vi "Main - Fan Characterisation - Dynamic - [Student].vi"() -> ()   [LabVIEW 2017]
uses:
  <vilib>/Utility/file.llb/Read Delimited Spreadsheet (DBL).vi
  <vilib>/Analysis/baseanly.llb/Mean (DBL).vi
  <vilib>/Utility/file.llb/Write To Spreadsheet File (DBL).vi
  <vilib>/Analysis/NI_AALPro.lvlib
  <vilib>/Analysis/NI_AALBase.lvlib
panel:
  out "Post Processed Output":dbl[][](graph)
  out "Run-Time Data":cluster{"f":dbl, dbl}(graph)
  out "Time (s)":dbl(slide) scale=0.0..10.0
  out "Load Cell Calibration Data":cluster{"Y":dbl[], "Y":dbl[]}[](graph)
  in  "stop":bool
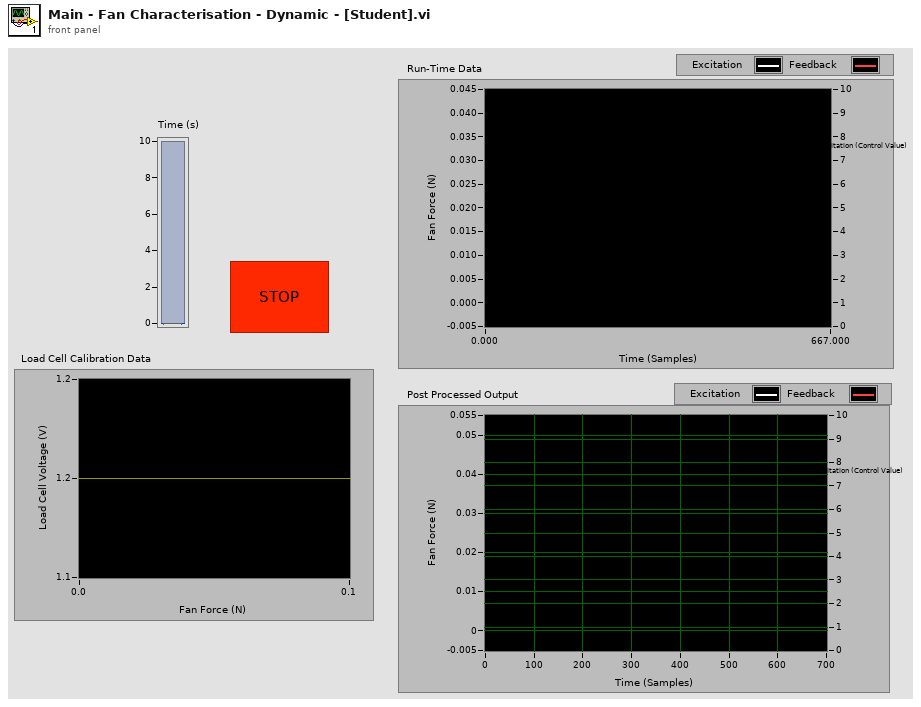
[diagram p1: front panel]
types:
  T1 = cluster{"AI Task":refnum<k21>, "Ctr0 Task":refnum<k21>, "Ao Task":refnum<k21>, "DO Task":refnum<k21>}
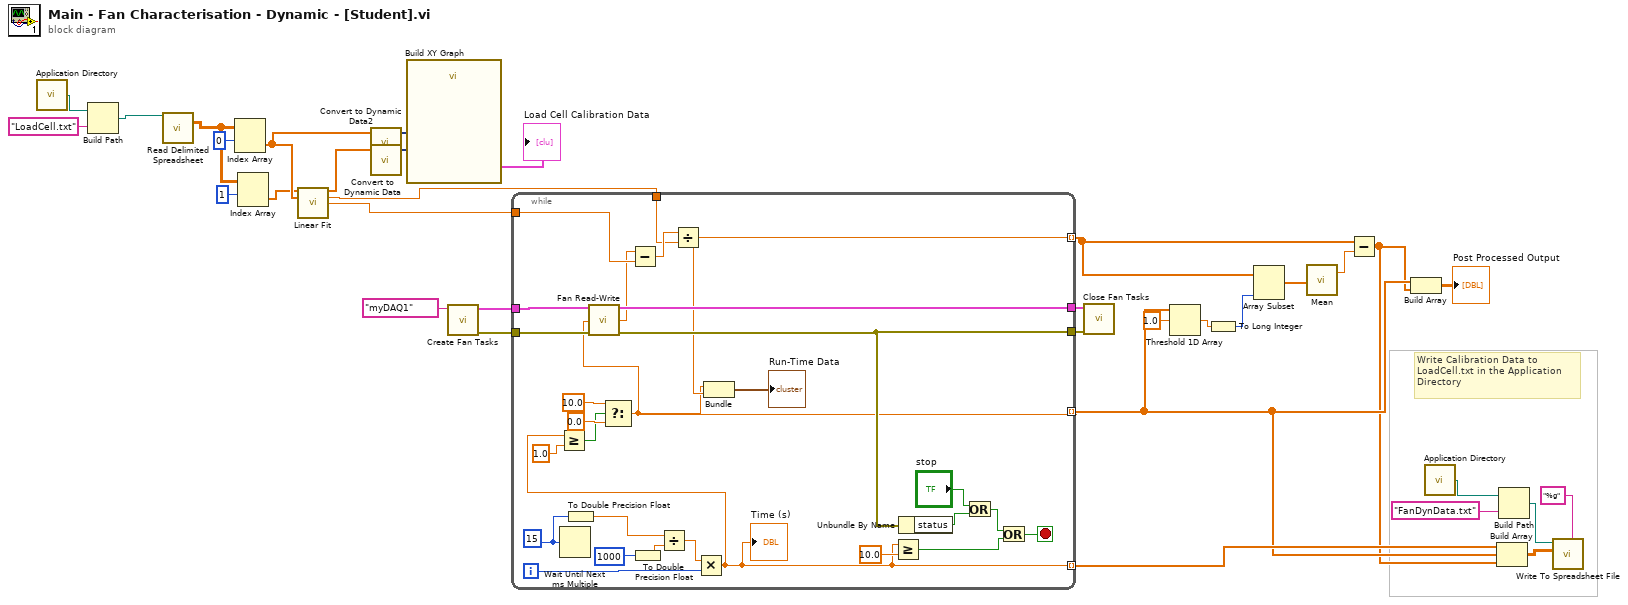
[diagram p0: block diagram]
diagram:
  # "Write Calibration Data to \nLoadCell.txt in the Application \nDirectory"
  n1 = call <vilib>:"Application Directory.vi"() -> ("Application Directory"=w23:path)
  n2 = Build Path(base path=w23, name or relative path="LoadCell.txt") -> (appended path=w22:path)
  n3 = call-poly <vilib>:"Read Delimited Spreadsheet.vi"("file path (dialog if empty)"=w22) -> ("all rows"=w25:dbl[][])  [unwired: 9 in, 5 out]
  n4 = Index Array(array=w25, index (row)=0) -> (element=w28:dbl[])  [unwired: 1 in]
  n5 = Index Array(array=w25, index (row)=1) -> (element=w26:dbl[])  [unwired: 1 in]
  n6 = call <vilib>:"Linear Fit.vi"("Y"=w26, "X"=w28) -> ("Best Linear Fit"=w16:dbl[], "slope"=w17:dbl, "intercept"=w18:dbl)  [unwired: 9 in, 2 out]
  n7 = call "Convert to Dynamic Data2"("Array"=w28) -> ("Dynamic Data Type"=w29:dynamicdata)  [unwired: 3 in]
  n8 = call "Convert to Dynamic Data"("Array"=w16) -> ("Dynamic Data Type"=w27:dynamicdata)  [unwired: 3 in]
  n9 = call "Build XY Graph"("Y Input"=w27, "X Input"=w29) -> ("XY Graph"=→"Load Cell Calibration Data":cluster{"X":dbl[], "Y":dbl[]}[])  [unwired: 8 in, 1 out]
  n10 = call "Create Fan Tasks.vi"("DAQmx Device Name"=tag "myDAQ1") -> ("Error Out"=w33:errorcluster, "Hellicopter Tasks Output"=w34:T1)  [unwired: 5 in]
  n11 = while {
    tunnel: w34 -> [w61]
    tunnel: w33 -> [w62]
    tunnel: [w60] -> w32
    tunnel: [w58] -> w31
    tunnel: w18 -> [w56]
    tunnel: w17 -> [w53]
    tunnel: [w35] -> w2 mode=indexing
    tunnel: [w38] -> w4 mode=indexing
    tunnel: [w36] -> w15 mode=indexing
    i -> [w52]
    stop <- w42 stop-if-true
    w47 = u32 15 ("millisecond multiple")
    n12 = Wait Until Next ms Multiple(millisecond multiple=w47) -> ()  [unwired: 1 out]
    n13 = To Double Precision Float(number=w47) -> (double precision float=w48:dbl)
    n14 = To Double Precision Float(number=u32 1000 ("y")) -> (double precision float=w49:dbl)
    n15 = Divide(x=w48, y=w49) -> (x/y=w51:dbl)
    n16 = Multiply(x=w51, y=w52) -> (x*y=w38:dbl)
    "Time (s)" <- w38
    n17 = Greater Or Equal?(x=w38, y=1.0) -> (x >= y?=w43:bool)
    n18 = Select(t=10.0, s=w43, f=0.0) -> (s? t:f=w35:dbl)
    n19 = call "Fan Read-Write.vi"("Hellicopter Tasks Input"=w61, "Fan Input"=w35, "Error In"=w62) -> ("Hellicopter Tasks Output"=w60:T1, "L/C Output"=w55:dbl, "Error Out"=w58:errorcluster)  [unwired: 10 in]
    n20 = Subtract(x=w55, y=w56) -> (x-y=w54:dbl)
    n21 = Divide(x=w54, y=w53) -> (x/y=w36:dbl)
    n22 = Bundle("f"=w35, w36) -> (→"Run-Time Data":cluster{"f":dbl, dbl})  [unwired: 1 in]
    n23 = Greater Or Equal?(x=w38, y=10.0) -> (x >= y?=w40:bool)
    n24 = Unbundle By Name(w58) -> ("status"=w57:bool)
    n25 = Or(x="stop", y=w57) -> (x .or. y?=w41:bool)
    n26 = Or(x=w41, y=w40) -> (x .or. y?=w42:bool)
  }
  n27 = call "Close Fan Tasks.vi"("Error In"=w31, "Hellicopter Tasks Input 2"=w32) -> ()  [unwired: 9 in, 1 out]
  n28 = Threshold 1D Array(2:1.0 ("threshold y"), 3:w2) -> (0:w10:dbl)  [unwired: 1 in]
  n29 = To Long Integer(number=w10) -> (32bit integer=w9:i32)
  n30 = Array Subset(array=w15, length=w9) -> (w14:dbl[])  [unwired: 1 in]
  n31 = call-poly <vilib>:"Mean.vi"("X"=w14) -> ("mean"=w13:dbl)  [unwired: 1 out]
  n32 = Subtract(x=w15, y=w13) -> (x-y=w1:dbl[])
  n33 = Build Array(w2, w1) -> (→"Post Processed Output":dbl[][])
  n34 = call <vilib>:"Application Directory.vi"() -> ("Application Directory"=w8:path)
  n35 = Build Array(w4, w2, w1) -> (w3:dbl[][])
  n36 = Build Path(base path=w8, name or relative path="FanDynData.txt") -> (appended path=w6:path)
  n37 = call-poly <vilib>:"Write To Spreadsheet File.vi"("format (%.3f)"="%g", "2D data"=w3, "file path (dialog if empty)"=w6) -> ()  [unwired: 5 in, 1 out]
